vi "Setup User Events.vi"(8 "error in (no error)":errorcluster, 9 "User Events in":refnum<class "UserEvents.lvclass">, 10 "Model in":refnum<class "Model.lvclass">, 11 "Boot Loader in":refnum<class "Boot Loader.lvclass">) -> (0 "error out":errorcluster, 1 "User Events out":refnum<class "UserEvents.lvclass">, 2 "Model out":refnum<class "Model.lvclass">, 3 "Boot Loader out":refnum<class "Boot Loader.lvclass">)   [LabVIEW 2015, in "Boot Loader.lvclass"]
uses:
  Boot Loader.lvclass
  Model/Model.lvclass
  UserEvents/UserEvents.lvclass
  Model/Model.lvclass/Model.ctl
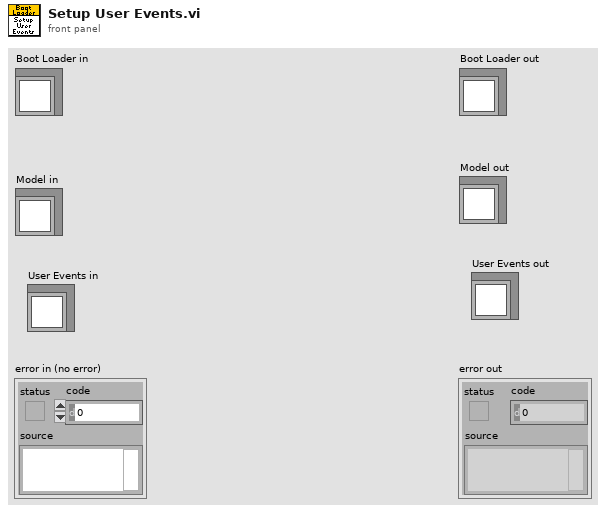
[diagram p1: front panel]
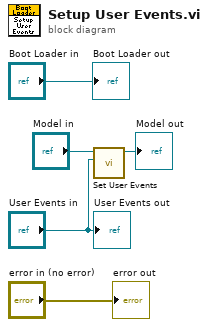
[diagram p0: block diagram]
diagram:
  n1 = call "Set User Events.vi"("userEvents"="User Events in", "Model in"="Model in") -> ("Model out"=→"Model out":refnum<class "Model.lvclass">)  [unwired: 9 in]
  "error out" <- "error in (no error)"
  "Boot Loader out" <- "Boot Loader in"
  "User Events out" <- "User Events in"
